vi "Main.vi"() -> ()   [LabVIEW 2017]
uses:
  <vilib>/Platform/TimedLoop/XDataNode/timing_clust.ctl
  <vilib>/Platform/TimedLoop/XDataNode/nitl_modes.ctl
  <vilib>/Platform/TimedLoop/XDataNode/wakeup.ctl
  <vilib>/Analysis/baseanly.llb/Mean (DBL).vi
  <vilib>/platform/TimedLoop/XDataNode/XDataNode.xnode
  <userlib>/dxl_x86_c/dxl_x86_c.lvlib
  <vilib>/Analysis/NI_AALBase.lvlib
  <vilib>/Platform/TimedLoop/XDataNode/XDNodeRunTimeDep.lvlib
panel:
  out "ADDR_MX_\nGOAL_POSITION":u16=30
  out "ADDR_MX_D":u16=26
  out "ADDR_MX_I":u16=27
  out "ADDR_MX_P":u16=28
  in  "PID gains":cluster{"Kp":dbl, "Ki":dbl, "Kd":dbl}={"Kp"=0.5, "Ki"=0.1, "Kd"=0.01} {"Kd" format="%.3f"; "Ki" format="%.3f"; "Kp" format="%.3f"}
  out "XY Graph":cluster{dbl[], dbl[]}(graph)={[0.0, 0.0, 21.21667205549289, 40.84932767864532, 14.13895464430464, 0.0], [0.0, 4.5, -15.269998150977838, -36.613822390853436, -25.31975437413041, 0.0]}
  in  "w":dbl=4.5
  in  "b 1":dbl=29.0
  in  "a 1":dbl=29.0
  out "theta 2":dbl=132.978515625
  out "theta 1":dbl=150.8203125
  out "delta load 2":dbl=0.09090909090908994
  out "value : MX\npresent speed 2":u16
  out "value : MX\npresent position 2":u16=2537
  out "value : MX\ngoal torque 2":u16
  out "value: MX\npresent load 2":u16=20
  in  "dynamixel_id 2":u8=11
  in  "locking ticks":i32=5
  in  "load trigger":dbl=40.0
  out "delta load 1":dbl=-2.8090909090909086
  out "value : MX\npresent speed 1":u16
  in  "torque 1 + torque 2":dbl=120.0
  out "CONTROL MODE":string="POSITION LOCK"
  out "value: MX\npresent load 1":u16=28
  out "ADDR_MX_\nPRESENT_LOAD":u16=40
  out "ADDR_MX_\nPRESENT_SPEED":u16=38
  out "ADDR_MX_\nTORQUE_CONTROL_MODE_ENABLE":u16=70
  out "value : MX\ngoal torque 1":u16
  in  "terminate":bool
  out "value : MX\npresent position 1":u16=2740
  out "baud_rate":i32=57600
  in  "dynamixel_id 1":u8=12
  out "protocol_version":dbl=1.0
  out "port_num":i32
  out "ADDR_MX_\nTORQUE_ENABLE":u16=24
  out "ADDR_MX_\nGOAL_TORQUE":u16=71
  out "ADDR_MX_\nPRESENT_POSITION":u16=36
  out "device_name":string="COM3"
  out "dynamixel_comm_result":string="[TxRxResult] Communication success."
  out "dynamixel_error":string
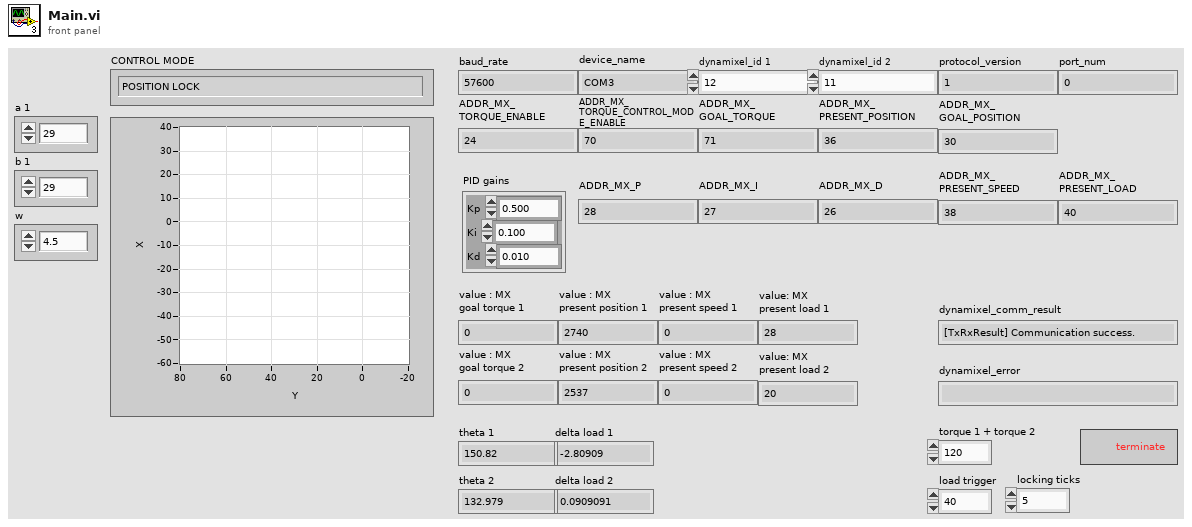
[diagram p1: front panel]
types:
  T1 = typedef "XDNodeRunTimeDep.lvlib/timing_clust.ctl" = cluster{"Expected End [f-1]":u64, "Actual End [f-1]":u64, "Finished Late? [f-1]":bool, "Expected End [i-1]":u64, "Actual End [i-1]":u64, "Finished Late? [i-1]":bool, "Expected Start [i]":u64, "Actual Start [i]":u64, "Expected Start [f]":u64, "Actual Start [f]":u64, "Source Name":string, "Structure Name":string, "Period":i64, "Deadline":i64, "Offset":i64, "Start":i64, "Priority":i32, "Timeout":i32, "Mode":T2, "Wakeup Reason":T3, "Error":errorcluster, "Source Type":string, "Secondary Source Type":string, "Global End Time":u64, "Global Start Time":u64, "Frame Duration":u64, "Iteration Duration":u64, "Assigned CPU":i32, "I/O Scan Engine Mode":u32}
  T2 = typedef "XDNodeRunTimeDep.lvlib/nitl_modes.ctl" = enum32{"No Change", "Process missed periods, maintain original phase", "Discard missed periods, maintain original phase", "Process missed periods, ignore original phase", "Discard missed periods, ignore original phase"}
  T3 = typedef "XDNodeRunTimeDep.lvlib/wakeup.ctl" = enum32{"Normal", "Aborted", "Asynchronous wakeup", "Timing source error", "Timed loop error", "Timeout"}
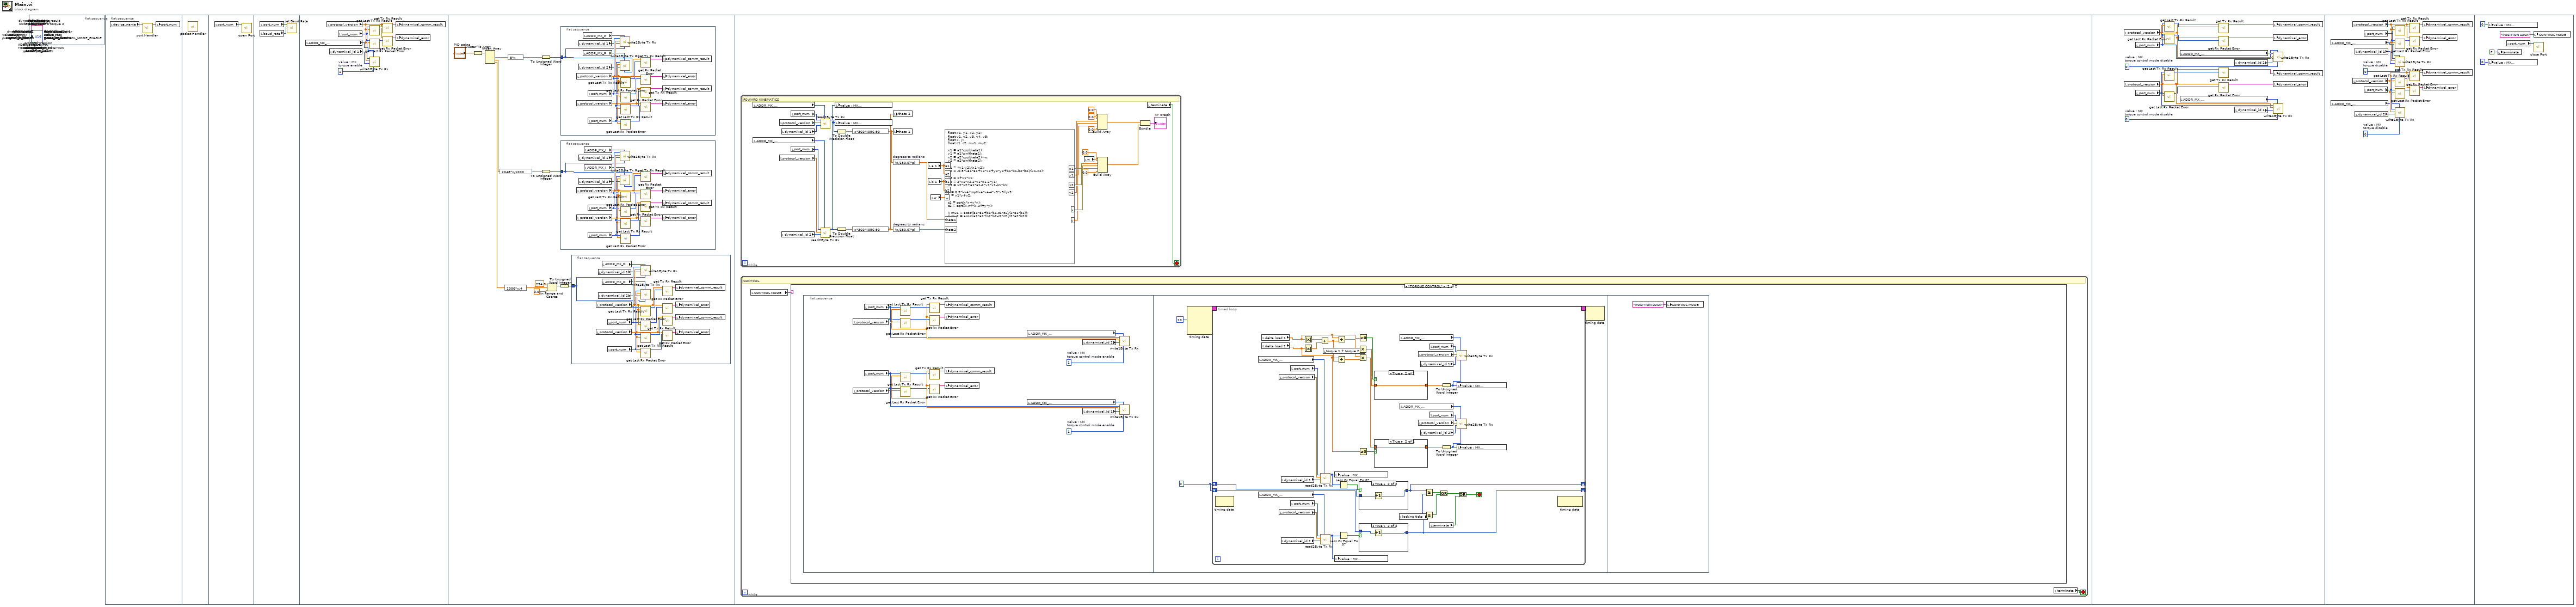
[diagram p0: block diagram]
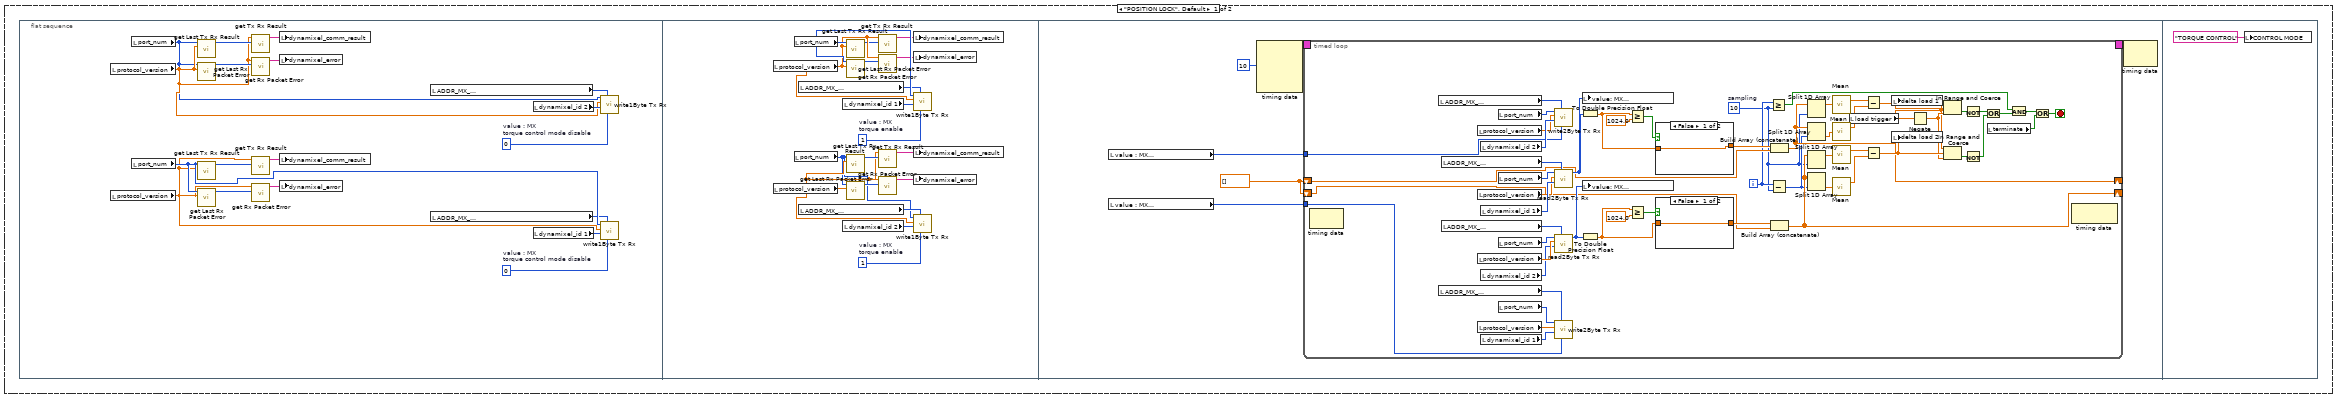
[diagram p2: hidden frame]
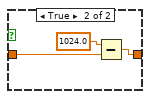
[diagram p3: hidden frame]
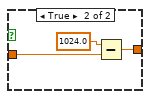
[diagram p4: hidden frame]
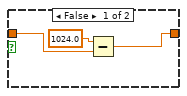
[diagram p5: hidden frame]
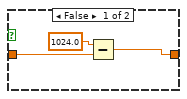
[diagram p6: hidden frame]
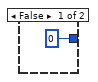
[diagram p7: hidden frame]
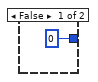
[diagram p8: hidden frame]
diagram:
  n1 = flat-sequence {
    frame #0 {
    }
  }
  n2 = flat-sequence {
    frame #0 {
      n3 = local read "device_name"() -> (w2:string)
      n4 = call <userlib>:"port Handler.vi"("port_name"=w2) -> ("function return"=w1:i32)  [unwired: 10 in]
      n5 = local write "port_num"(w1) -> ()
    }
    frame #1 {
      n6 = call <userlib>:"packet Handler.vi"() -> ()  [unwired: 12 in]
    }
    frame #2 {
      n7 = local read "port_num"() -> (w3:i32)
      n8 = call <userlib>:"open Port.vi"("port_num"=w3) -> ()  [unwired: 10 in, 1 out]
    }
    frame #3 {
      n9 = local read "port_num"() -> (w4:i32)
      n10 = local read "baud_rate"() -> (w5:i32)
      n11 = call <userlib>:"set Baud Rate.vi"("baudrate"=w5, "port_num"=w4) -> ()  [unwired: 9 in, 1 out]
    }
    frame #4 {
      w7 = 1  # value : MX torque enable
      n12 = local read "ADDR_MX_\nTORQUE_ENABLE"() -> (w14:u16)
      n13 = local read "protocol_version"() -> (w6:dbl)
      n14 = local read "dynamixel_id 1"() -> (w13:u8)
      n15 = local read "port_num"() -> (w8:i32)
      n16 = call <userlib>:"get Last Tx Rx Result.vi"("protocol_version"=w6, "port_num"=w8) -> ("function return"=w9:i32)  [unwired: 9 in]
      n17 = call <userlib>:"get Last Rx Packet Error.vi"("protocol_version"=w6, "port_num"=w8) -> ("function return"=w10:u8)  [unwired: 9 in]
      n18 = call <userlib>:"write1Byte Tx Rx.vi"("data"=w7, "address"=w14, "id"=w13, "protocol_version"=w6, "port_num"=w8) -> ()  [unwired: 7 in]
      n19 = call <userlib>:"get Tx Rx Result.vi"("result"=w9, "protocol_version"=w6) -> ("function return"=w11:string)  [unwired: 9 in]
      n20 = call <userlib>:"get Rx Packet Error.vi"("error"=w10, "protocol_version"=w6) -> ("function return"=w12:string)  [unwired: 9 in]
      n21 = local write "dynamixel_comm_result"(w11) -> ()
      n22 = local write "dynamixel_error"(w12) -> ()
    }
    frame #5 {
      n23 = Cluster To Array(cluster="PID gains") -> (array=w27:dbl[])
      n24 = Index Array(array=w27) -> (element #1=w26:dbl, element #2=w25:dbl, element #3=w24:dbl)  [unwired: 3 in]
      n25 = expression code="2048*x/1000"(w25) -> (w22:dbl)
      n26 = expression code="1000*x/4"(w24) -> (w19:dbl)
      n27 = expression code="8*x"(w26) -> (w23:dbl)
      n28 = To Unsigned Word Integer(number=w23) -> (unsigned 16bit integer=w17:u16)
      n29 = To Unsigned Word Integer(number=w22) -> (unsigned 16bit integer=w16:u16)
      n30 = In Range and Coerce(upper limit=254.0, x=w19, lower limit=0.0) -> (coerced(x)=w18:dbl)  [unwired: 1 out]
      n31 = To Unsigned Word Integer(number=w18) -> (unsigned 16bit integer=w15:u16)
      n32 = flat-sequence {
        tunnel: w17 -> [w63]
        frame #0 {
          n33 = local read "protocol_version"() -> (w79:dbl)
          n34 = local read "protocol_version"() -> (w64:dbl)
          n35 = local read "dynamixel_id 1"() -> (w73:u8)
          n36 = local read "dynamixel_id 2"() -> (w70:u8)
          n37 = local read "ADDR_MX_P"() -> (w72:u16)
          n38 = local read "ADDR_MX_P"() -> (w71:u16)
          n39 = local read "port_num"() -> (w78:i32)
          n40 = local read "port_num"() -> (w65:i32)
          n41 = call <userlib>:"write1Byte Tx Rx.vi"("data"=w63, "address"=w72, "id"=w73, "protocol_version"=w79, "port_num"=w78) -> ()  [unwired: 7 in]
          n42 = call <userlib>:"write1Byte Tx Rx.vi"("data"=w63, "address"=w71, "id"=w70, "protocol_version"=w64, "port_num"=w65) -> ()  [unwired: 7 in]
          n43 = call <userlib>:"get Last Tx Rx Result.vi"("protocol_version"=w79, "port_num"=w78) -> ("function return"=w77:i32)  [unwired: 9 in]
          n44 = call <userlib>:"get Last Rx Packet Error.vi"("protocol_version"=w79, "port_num"=w78) -> ("function return"=w76:u8)  [unwired: 9 in]
          n45 = call <userlib>:"get Last Tx Rx Result.vi"("protocol_version"=w64, "port_num"=w65) -> ("function return"=w66:i32)  [unwired: 9 in]
          n46 = call <userlib>:"get Last Rx Packet Error.vi"("protocol_version"=w64, "port_num"=w65) -> ("function return"=w67:u8)  [unwired: 9 in]
          n47 = call <userlib>:"get Tx Rx Result.vi"("result"=w77, "protocol_version"=w79) -> ("function return"=w75:string)  [unwired: 9 in]
          n48 = call <userlib>:"get Rx Packet Error.vi"("error"=w76, "protocol_version"=w79) -> ("function return"=w74:string)  [unwired: 9 in]
          n49 = call <userlib>:"get Tx Rx Result.vi"("result"=w66, "protocol_version"=w64) -> ("function return"=w68:string)  [unwired: 9 in]
          n50 = call <userlib>:"get Rx Packet Error.vi"("error"=w67, "protocol_version"=w64) -> ("function return"=w69:string)  [unwired: 9 in]
          n51 = local write "dynamixel_comm_result"(w75) -> ()
          n52 = local write "dynamixel_error"(w74) -> ()
          n53 = local write "dynamixel_comm_result"(w68) -> ()
          n54 = local write "dynamixel_error"(w69) -> ()
        }
      }
      n55 = flat-sequence {
        tunnel: w16 -> [w46]
        frame #0 {
          n56 = local read "protocol_version"() -> (w62:dbl)
          n57 = local read "protocol_version"() -> (w47:dbl)
          n58 = local read "dynamixel_id 1"() -> (w56:u8)
          n59 = local read "dynamixel_id 2"() -> (w53:u8)
          n60 = local read "ADDR_MX_I"() -> (w55:u16)
          n61 = local read "ADDR_MX_I"() -> (w54:u16)
          n62 = local read "port_num"() -> (w61:i32)
          n63 = local read "port_num"() -> (w48:i32)
          n64 = call <userlib>:"write1Byte Tx Rx.vi"("data"=w46, "address"=w55, "id"=w56, "protocol_version"=w62, "port_num"=w61) -> ()  [unwired: 7 in]
          n65 = call <userlib>:"write1Byte Tx Rx.vi"("data"=w46, "address"=w54, "id"=w53, "protocol_version"=w47, "port_num"=w48) -> ()  [unwired: 7 in]
          n66 = call <userlib>:"get Last Tx Rx Result.vi"("protocol_version"=w62, "port_num"=w61) -> ("function return"=w60:i32)  [unwired: 9 in]
          n67 = call <userlib>:"get Last Rx Packet Error.vi"("protocol_version"=w62, "port_num"=w61) -> ("function return"=w59:u8)  [unwired: 9 in]
          n68 = call <userlib>:"get Last Tx Rx Result.vi"("protocol_version"=w47, "port_num"=w48) -> ("function return"=w49:i32)  [unwired: 9 in]
          n69 = call <userlib>:"get Last Rx Packet Error.vi"("protocol_version"=w47, "port_num"=w48) -> ("function return"=w50:u8)  [unwired: 9 in]
          n70 = call <userlib>:"get Tx Rx Result.vi"("result"=w60, "protocol_version"=w62) -> ("function return"=w58:string)  [unwired: 9 in]
          n71 = call <userlib>:"get Rx Packet Error.vi"("error"=w59, "protocol_version"=w62) -> ("function return"=w57:string)  [unwired: 9 in]
          n72 = call <userlib>:"get Tx Rx Result.vi"("result"=w49, "protocol_version"=w47) -> ("function return"=w51:string)  [unwired: 9 in]
          n73 = call <userlib>:"get Rx Packet Error.vi"("error"=w50, "protocol_version"=w47) -> ("function return"=w52:string)  [unwired: 9 in]
          n74 = local write "dynamixel_comm_result"(w58) -> ()
          n75 = local write "dynamixel_error"(w57) -> ()
          n76 = local write "dynamixel_comm_result"(w51) -> ()
          n77 = local write "dynamixel_error"(w52) -> ()
        }
      }
      n78 = flat-sequence {
        tunnel: w15 -> [w29]
        frame #0 {
          n79 = local read "protocol_version"() -> (w45:dbl)
          n80 = local read "protocol_version"() -> (w30:dbl)
          n81 = local read "dynamixel_id 1"() -> (w39:u8)
          n82 = local read "dynamixel_id 2"() -> (w36:u8)
          n83 = local read "ADDR_MX_D"() -> (w38:u16)
          n84 = local read "ADDR_MX_D"() -> (w37:u16)
          n85 = local read "port_num"() -> (w44:i32)
          n86 = local read "port_num"() -> (w31:i32)
          n87 = call <userlib>:"write1Byte Tx Rx.vi"("data"=w29, "address"=w38, "id"=w39, "protocol_version"=w45, "port_num"=w44) -> ()  [unwired: 7 in]
          n88 = call <userlib>:"write1Byte Tx Rx.vi"("data"=w29, "address"=w37, "id"=w36, "protocol_version"=w30, "port_num"=w31) -> ()  [unwired: 7 in]
          n89 = call <userlib>:"get Last Tx Rx Result.vi"("protocol_version"=w45, "port_num"=w44) -> ("function return"=w43:i32)  [unwired: 9 in]
          n90 = call <userlib>:"get Last Rx Packet Error.vi"("protocol_version"=w45, "port_num"=w44) -> ("function return"=w42:u8)  [unwired: 9 in]
          n91 = call <userlib>:"get Last Tx Rx Result.vi"("protocol_version"=w30, "port_num"=w31) -> ("function return"=w32:i32)  [unwired: 9 in]
          n92 = call <userlib>:"get Last Rx Packet Error.vi"("protocol_version"=w30, "port_num"=w31) -> ("function return"=w33:u8)  [unwired: 9 in]
          n93 = call <userlib>:"get Tx Rx Result.vi"("result"=w43, "protocol_version"=w45) -> ("function return"=w41:string)  [unwired: 9 in]
          n94 = call <userlib>:"get Rx Packet Error.vi"("error"=w42, "protocol_version"=w45) -> ("function return"=w40:string)  [unwired: 9 in]
          n95 = call <userlib>:"get Tx Rx Result.vi"("result"=w32, "protocol_version"=w30) -> ("function return"=w34:string)  [unwired: 9 in]
          n96 = call <userlib>:"get Rx Packet Error.vi"("error"=w33, "protocol_version"=w30) -> ("function return"=w35:string)  [unwired: 9 in]
          n97 = local write "dynamixel_comm_result"(w41) -> ()
          n98 = local write "dynamixel_error"(w40) -> ()
          n99 = local write "dynamixel_comm_result"(w34) -> ()
          n100 = local write "dynamixel_error"(w35) -> ()
        }
      }
    }
    frame #6 {
      n101 = while {
        stop <- w81 stop-if-true
        # "FOWARD KINEMATICS"
        n102 = local read "ADDR_MX_\nPRESENT_POSITION"() -> (w114:u16)
        n103 = local read "ADDR_MX_\nPRESENT_POSITION"() -> (w107:u16)
        n104 = local read "protocol_version"() -> (w112:dbl)
        n105 = local read "protocol_version"() -> (w109:dbl)
        n106 = local read "dynamixel_id 1"() -> (w111:u8)
        n107 = local read "dynamixel_id 2"() -> (w110:u8)
        n108 = local read "port_num"() -> (w113:i32)
        n109 = local read "port_num"() -> (w108:i32)
        n110 = call <userlib>:"read2Byte Tx Rx.vi"("address"=w114, "id"=w111, "protocol_version"=w112, "port_num"=w113) -> ("function return"=w106:u16)  [unwired: 7 in]
        n111 = call <userlib>:"read2Byte Tx Rx.vi"("address"=w107, "id"=w110, "protocol_version"=w109, "port_num"=w108) -> ("function return"=w104:u16)  [unwired: 7 in]
        n112 = local write "value : MX\npresent position 2"(w104) -> ()
        n113 = local write "value : MX\npresent position 1"(w106) -> ()
        n114 = To Double Precision Float(number=w106) -> (double precision float=w105:dbl)
        n115 = To Double Precision Float(number=w104) -> (double precision float=w103:dbl)
        n116 = expression code="x*360/4096-90"(w105) -> (w88:dbl)
        n117 = expression code="x*360/4096-90"(w103) -> (w90:dbl)
        n118 = local write "theta 2"(w90) -> ()
        n119 = local write "theta 1"(w88) -> ()
        n120 = expression code="(x/180.0)*pi" "degrees to radians"(w88) -> (w87:dbl)
        n121 = expression code="(x/180.0)*pi" "degrees to radians"(w90) -> (w89:dbl)
        n122 = local read "a 1"() -> (w102:dbl)
        n123 = local read "b 1"() -> (w100:dbl)
        n124 = local read "w"() -> (w101:dbl)
        n125 = formula code="float x1, y1, x2, y2;\nfloat v1, v2, v3, v4, v5;\nfloat x, y;\nfloat c1, c2, mu1, mu2;\n\nx1 = a1*cos(theta1);\ny1 = a1*sin(theta1);\nx2 = a2*cos(theta2)+w;\ny2 = a2*sin(theta2);\n\nv1 = -(y1-y2)/(x1-x2);\nv2 = -0.5*(-a1*a1+x2*x2+y2*y2+b1*b1-b2*b2)/(x1-x2);\n\nv3 = 1+v1*v1;\nv4 = 2*v1*v2-2*v1*x1-2*y1;\nv5 = v2*v2+a1*a1-2*v2*x1-b1*b1;\n\ny = 0.5*(-v4+sqrt(v4*v4-4*v3*v5))/v3;\nx = v1*y+v2;\n\nc1 = sqrt(x*x+y*y);\nc2 = sqrt((x-w)*(x-w)+y*y);\n\n// mu1 = acos((a1*a1+b1*b1-c1*c1)/(2*a1*b1));\n// mu2 = acos((a2*a2+b2*b2-c2*c2)/(2*a2*b2));"("a1"=w102, "a2"=w102, "b1"=w100, "b2"=w100, "w"=w101, "theta1"=w87, "theta2"=w89) -> ("x1"=w96:dbl, "y1"=w93:dbl, "x2"=w98:dbl, "y2"=w95:dbl, "x"=w97:dbl, "y"=w94:dbl)
        n126 = local read "w"() -> (w99:dbl)
        n127 = Build Array(0.0 ("element"), 0.0 ("element"), w95, w94, w93, 0.0 ("element")) -> (w91:dbl[])
        n128 = Build Array(0.0 ("element"), w99, w98, w97, w96, 0.0 ("element")) -> (w92:dbl[])
        n129 = Bundle(w91, w92) -> (→"XY Graph":cluster{dbl[], dbl[]})  [unwired: 1 in]
        n130 = local read "terminate"() -> (w81:bool)
      }
      n131 = while {
        stop <- w116 stop-if-true
        # "CONTROL"
        n132 = local read "CONTROL MODE"() -> (w115:string)
        n133 = case shown="\"TORQUE CONTROL\"" w115 {
          frame "POSITION LOCK", Default {
            n134 = flat-sequence {
              frame #0 {
                w117 = 0  # value : MX torque control mode disable
                w134 = 0  # value : MX torque control mode disable
                n135 = local read "protocol_version"() -> (w119:dbl)
                n136 = local read "protocol_version"() -> (w132:dbl)
                n137 = local read "port_num"() -> (w118:i32)
                n138 = local read "port_num"() -> (w133:i32)
                n139 = call <userlib>:"get Last Tx Rx Result.vi"("protocol_version"=w119, "port_num"=w118) -> ("function return"=w120:i32)  [unwired: 9 in]
                n140 = call <userlib>:"get Last Rx Packet Error.vi"("protocol_version"=w119, "port_num"=w118) -> ("function return"=w121:u8)  [unwired: 9 in]
                n141 = call <userlib>:"get Last Tx Rx Result.vi"("protocol_version"=w132, "port_num"=w133) -> ("function return"=w131:i32)  [unwired: 9 in]
                n142 = call <userlib>:"get Last Rx Packet Error.vi"("protocol_version"=w132, "port_num"=w133) -> ("function return"=w130:u8)  [unwired: 9 in]
                n143 = call <userlib>:"get Tx Rx Result.vi"("result"=w120, "protocol_version"=w119) -> ("function return"=w122:string)  [unwired: 9 in]
                n144 = call <userlib>:"get Rx Packet Error.vi"("error"=w121, "protocol_version"=w119) -> ("function return"=w123:string)  [unwired: 9 in]
                n145 = call <userlib>:"get Tx Rx Result.vi"("result"=w131, "protocol_version"=w132) -> ("function return"=w129:string)  [unwired: 9 in]
                n146 = call <userlib>:"get Rx Packet Error.vi"("error"=w130, "protocol_version"=w132) -> ("function return"=w128:string)  [unwired: 9 in]
                n147 = local write "dynamixel_comm_result"(w122) -> ()
                n148 = local write "dynamixel_error"(w123) -> ()
                n149 = local write "dynamixel_comm_result"(w129) -> ()
                n150 = local write "dynamixel_error"(w128) -> ()
                n151 = local read "ADDR_MX_\nTORQUE_CONTROL_MODE_ENABLE"() -> (w125:u16)
                n152 = local read "ADDR_MX_\nTORQUE_CONTROL_MODE_ENABLE"() -> (w126:u16)
                n153 = local read "dynamixel_id 2"() -> (w124:u8)
                n154 = local read "dynamixel_id 1"() -> (w127:u8)
                n155 = call <userlib>:"write1Byte Tx Rx.vi"("data"=w117, "address"=w125, "id"=w124, "protocol_version"=w119, "port_num"=w118) -> ()  [unwired: 7 in]
                n156 = call <userlib>:"write1Byte Tx Rx.vi"("data"=w134, "address"=w126, "id"=w127, "protocol_version"=w132, "port_num"=w133) -> ()  [unwired: 7 in]
              }
              frame #1 {
                w135 = 1  # value : MX torque enable
                w152 = 1  # value : MX torque enable
                n157 = local read "protocol_version"() -> (w150:dbl)
                n158 = local read "protocol_version"() -> (w137:dbl)
                n159 = local read "port_num"() -> (w151:i32)
                n160 = local read "port_num"() -> (w136:i32)
                n161 = local read "ADDR_MX_\nTORQUE_ENABLE"() -> (w144:u16)
                n162 = local read "ADDR_MX_\nTORQUE_ENABLE"() -> (w143:u16)
                n163 = local read "dynamixel_id 1"() -> (w145:u8)
                n164 = local read "dynamixel_id 2"() -> (w142:u8)
                n165 = call <userlib>:"get Last Tx Rx Result.vi"("protocol_version"=w150, "port_num"=w151) -> ("function return"=w149:i32)  [unwired: 9 in]
                n166 = call <userlib>:"get Last Rx Packet Error.vi"("protocol_version"=w150, "port_num"=w151) -> ("function return"=w148:u8)  [unwired: 9 in]
                n167 = call <userlib>:"get Last Tx Rx Result.vi"("protocol_version"=w137, "port_num"=w136) -> ("function return"=w138:i32)  [unwired: 9 in]
                n168 = call <userlib>:"get Last Rx Packet Error.vi"("protocol_version"=w137, "port_num"=w136) -> ("function return"=w139:u8)  [unwired: 9 in]
                n169 = call <userlib>:"get Tx Rx Result.vi"("result"=w149, "protocol_version"=w150) -> ("function return"=w147:string)  [unwired: 9 in]
                n170 = call <userlib>:"get Rx Packet Error.vi"("error"=w148, "protocol_version"=w150) -> ("function return"=w146:string)  [unwired: 9 in]
                n171 = call <userlib>:"get Tx Rx Result.vi"("result"=w138, "protocol_version"=w137) -> ("function return"=w140:string)  [unwired: 9 in]
                n172 = call <userlib>:"get Rx Packet Error.vi"("error"=w139, "protocol_version"=w137) -> ("function return"=w141:string)  [unwired: 9 in]
                n173 = local write "dynamixel_comm_result"(w147) -> ()
                n174 = local write "dynamixel_error"(w146) -> ()
                n175 = call <userlib>:"write1Byte Tx Rx.vi"("data"=w152, "address"=w144, "id"=w145, "protocol_version"=w150, "port_num"=w151) -> ()  [unwired: 7 in]
                n176 = local write "dynamixel_comm_result"(w140) -> ()
                n177 = local write "dynamixel_error"(w141) -> ()
                n178 = call <userlib>:"write1Byte Tx Rx.vi"("data"=w135, "address"=w143, "id"=w142, "protocol_version"=w137, "port_num"=w136) -> ()  [unwired: 7 in]
              }
              frame #2 {
                w155 = dbl[] []
                n179 = local read "value : MX\npresent position 2"() -> (w154:u16)
                n180 = local read "value : MX\npresent position 1"() -> (w153:u16)
                n181 = node-c288(i64 10 ("Period")) -> (w158:T1)  [unwired: 3 in]
                n182 = timed-loop {
                  shift-right: [w180] -> _
                  shift-left: w155 -> [w206]
                  shift-right: [w185] -> _
                  shift-left: w155 -> [w191]
                  timing: w158 -> [_]
                  timing-out: [_] -> w157
                  tunnel: w154 -> [w160]
                  tunnel: w153 -> [w159]
                  i -> [w173]
                  stop <- w188 stop-if-true
                  w172 = 10  # sampling
                  n183 = node-c288() -> ()  [unwired: 1 in, 1 out]
                  n184 = local read "ADDR_MX_\nGOAL_POSITION"() -> (w164:u16)
                  n185 = local read "ADDR_MX_\nGOAL_POSITION"() -> (w165:u16)
                  n186 = local read "ADDR_MX_\nPRESENT_LOAD"() -> (w214:u16)
                  n187 = local read "ADDR_MX_\nPRESENT_LOAD"() -> (w192:u16)
                  n188 = local read "protocol_version"() -> (w162:dbl)
                  n189 = local read "protocol_version"() -> (w211:dbl)
                  n190 = local read "protocol_version"() -> (w195:dbl)
                  n191 = local read "protocol_version"() -> (w167:dbl)
                  n192 = local read "dynamixel_id 2"() -> (w163:u8)
                  n193 = local read "dynamixel_id 1"() -> (w212:u8)
                  n194 = local read "dynamixel_id 2"() -> (w194:u8)
                  n195 = local read "dynamixel_id 1"() -> (w166:u8)
                  n196 = local read "port_num"() -> (w161:i32)
                  n197 = local read "port_num"() -> (w213:i32)
                  n198 = local read "port_num"() -> (w193:i32)
                  n199 = local read "port_num"() -> (w168:i32)
                  n200 = call <userlib>:"write2Byte Tx Rx.vi"("data"=w160, "address"=w164, "id"=w163, "protocol_version"=w162, "port_num"=w161) -> ()  [unwired: 7 in]
                  n201 = call <userlib>:"read2Byte Tx Rx.vi"("address"=w214, "id"=w212, "protocol_version"=w211, "port_num"=w213) -> ("function return"=w207:u16)  [unwired: 7 in]
                  n202 = call <userlib>:"read2Byte Tx Rx.vi"("address"=w192, "id"=w194, "protocol_version"=w195, "port_num"=w193) -> ("function return"=w199:u16)  [unwired: 7 in]
                  n203 = call <userlib>:"write2Byte Tx Rx.vi"("data"=w159, "address"=w165, "id"=w166, "protocol_version"=w167, "port_num"=w168) -> ()  [unwired: 7 in]
                  n204 = To Double Precision Float(number=w207) -> (double precision float=w208:dbl)
                  n205 = To Double Precision Float(number=w199) -> (double precision float=w198:dbl)
                  n206 = local write "value: MX\npresent load 1"(w207) -> ()
                  n207 = local write "value: MX\npresent load 2"(w199) -> ()
                  n208 = Greater Or Equal?(x=w208, y=1024.0) -> (x >= y?=w209:bool)
                  n209 = Greater Or Equal?(x=w198, y=1024.0) -> (x >= y?=w197:bool)
                  n210 = case shown="False" w209 {
                    tunnel: w208 -> [w221 w223]
                    tunnel: [w221 w222] -> w204
                    frame False {
                    }
                    frame True {
                      n211 = Subtract(x=1024.0, y=w223) -> (x-y=w222:dbl)
                    }
                  }
                  n212 = case shown="False" w197 {
                    tunnel: w198 -> [w217 w219]
                    tunnel: [w217 w218] -> w201
                    frame False {
                    }
                    frame True {
                      n213 = Subtract(x=1024.0, y=w219) -> (x-y=w218:dbl)
                    }
                  }
                  n214 = Greater Or Equal?(x=w173, y=w172) -> (x >= y?=w174:bool)
                  n215 = Subtract(x=w173, y=w172) -> (x-y=w179:i32)
                  n216 = Build Array (concatenate)(w204, w206) -> (w180:dbl[])
                  n217 = Build Array (concatenate)(w201, w191) -> (w185:dbl[])
                  n218 = Split 1D Array(array=w180, index=w172) -> (first subarray=w205:dbl[])  [unwired: 1 out]
                  n219 = Split 1D Array(array=w180, index=w179) -> (second subarray=w181:dbl[])  [unwired: 1 out]
                  n220 = Split 1D Array(array=w185, index=w172) -> (first subarray=w200:dbl[])  [unwired: 1 out]
                  n221 = Split 1D Array(array=w185, index=w179) -> (second subarray=w186:dbl[])  [unwired: 1 out]
                  n222 = call-poly <vilib>:"Mean.vi"("X"=w205) -> ("mean"=w178:dbl)  [unwired: 1 out]
                  n223 = call-poly <vilib>:"Mean.vi"("X"=w181) -> ("mean"=w177:dbl)  [unwired: 1 out]
                  n224 = call-poly <vilib>:"Mean.vi"("X"=w200) -> ("mean"=w184:dbl)  [unwired: 1 out]
                  n225 = call-poly <vilib>:"Mean.vi"("X"=w186) -> ("mean"=w183:dbl)  [unwired: 1 out]
                  n226 = local read "load trigger"() -> (w169:dbl)
                  n227 = Subtract(x=w178, y=w177) -> (x-y=w176:dbl)
                  n228 = Subtract(x=w184, y=w183) -> (x-y=w182:dbl)
                  n229 = local write "delta load 1"(w176) -> ()
                  n230 = local write "delta load 2"(w182) -> ()
                  n231 = Negate(x=w169) -> (-x=w170:dbl)
                  n232 = In Range and Coerce(upper limit=w169, x=w176, lower limit=w170) -> (In Range?=w203:bool)  [unwired: 1 out]
                  n233 = In Range and Coerce(upper limit=w169, x=w182, lower limit=w170) -> (In Range?=w202:bool)  [unwired: 1 out]
                  n234 = Not(x=w203) -> (.not. x?=w187:bool)
                  n235 = Not(x=w202) -> (.not. x?=w190:bool)
                  n236 = Or(x=w187, y=w190) -> (x .or. y?=w175:bool)
                  n237 = local read "terminate"() -> (w189:bool)
                  n238 = And(x=w174, y=w175) -> (x .and. y?=w171:bool)
                  n239 = Or(x=w171, y=w189) -> (x .or. y?=w188:bool)
                  n240 = node-c288() -> ()  [unwired: 1 in, 1 out]
                }
                n241 = node-c288(w157) -> ()  [unwired: 1 out]
              }
              frame #3 {
                n242 = local write "CONTROL MODE"("TORQUE CONTROL" ("mode")) -> ()
              }
            }
          }
          frame "TORQUE CONTROL" {
            n243 = flat-sequence {
              frame #0 {
                w238 = 1  # value : MX torque control mode enable
                w239 = 1  # value : MX torque control mode enable
                n244 = local read "protocol_version"() -> (w231:dbl)
                n245 = local read "protocol_version"() -> (w246:dbl)
                n246 = local read "port_num"() -> (w230:i32)
                n247 = local read "port_num"() -> (w247:i32)
                n248 = call <userlib>:"get Last Tx Rx Result.vi"("protocol_version"=w231, "port_num"=w230) -> ("function return"=w232:i32)  [unwired: 9 in]
                n249 = call <userlib>:"get Last Rx Packet Error.vi"("protocol_version"=w231, "port_num"=w230) -> ("function return"=w233:u8)  [unwired: 9 in]
                n250 = call <userlib>:"get Last Tx Rx Result.vi"("protocol_version"=w246, "port_num"=w247) -> ("function return"=w245:i32)  [unwired: 9 in]
                n251 = call <userlib>:"get Last Rx Packet Error.vi"("protocol_version"=w246, "port_num"=w247) -> ("function return"=w244:u8)  [unwired: 9 in]
                n252 = call <userlib>:"get Tx Rx Result.vi"("result"=w232, "protocol_version"=w231) -> ("function return"=w234:string)  [unwired: 9 in]
                n253 = call <userlib>:"get Rx Packet Error.vi"("error"=w233, "protocol_version"=w231) -> ("function return"=w235:string)  [unwired: 9 in]
                n254 = call <userlib>:"get Tx Rx Result.vi"("result"=w245, "protocol_version"=w246) -> ("function return"=w243:string)  [unwired: 9 in]
                n255 = call <userlib>:"get Rx Packet Error.vi"("error"=w244, "protocol_version"=w246) -> ("function return"=w242:string)  [unwired: 9 in]
                n256 = local write "dynamixel_comm_result"(w234) -> ()
                n257 = local write "dynamixel_error"(w235) -> ()
                n258 = local write "dynamixel_comm_result"(w243) -> ()
                n259 = local write "dynamixel_error"(w242) -> ()
                n260 = local read "ADDR_MX_\nTORQUE_CONTROL_MODE_ENABLE"() -> (w237:u16)
                n261 = local read "ADDR_MX_\nTORQUE_CONTROL_MODE_ENABLE"() -> (w240:u16)
                n262 = local read "dynamixel_id 2"() -> (w236:u8)
                n263 = local read "dynamixel_id 1"() -> (w241:u8)
                n264 = call <userlib>:"write1Byte Tx Rx.vi"("data"=w238, "address"=w237, "id"=w236, "protocol_version"=w231, "port_num"=w230) -> ()  [unwired: 7 in]
                n265 = call <userlib>:"write1Byte Tx Rx.vi"("data"=w239, "address"=w240, "id"=w241, "protocol_version"=w246, "port_num"=w247) -> ()  [unwired: 7 in]
              }
              frame #1 {
                w251 = 0
                n266 = node-c288(i64 10 ("Period")) -> (w250:T1)  [unwired: 3 in]
                n267 = timed-loop {
                  shift-right: [w288] -> _
                  shift-left: w251 -> [w289]
                  shift-right: [w277] -> _
                  shift-left: w251 -> [w281]
                  timing: w250 -> [_]
                  timing-out: [_] -> w249
                  stop <- w291 stop-if-true
                  n268 = node-c288() -> ()  [unwired: 1 in, 1 out]
                  n269 = local read "ADDR_MX_\nPRESENT_SPEED"() -> (w297:u16)
                  n270 = local read "ADDR_MX_\nPRESENT_SPEED"() -> (w282:u16)
                  n271 = local read "delta load 1"() -> (w253:dbl)
                  n272 = local read "delta load 2"() -> (w252:dbl)
                  n273 = local read "protocol_version"() -> (w294:dbl)
                  n274 = local read "protocol_version"() -> (w285:dbl)
                  n275 = local read "dynamixel_id 1"() -> (w295:u8)
                  n276 = local read "dynamixel_id 2"() -> (w284:u8)
                  n277 = local read "port_num"() -> (w296:i32)
                  n278 = local read "port_num"() -> (w283:i32)
                  n279 = Absolute Value(x=w253) -> (abs(x)=w260:dbl)
                  n280 = Absolute Value(x=w252) -> (abs(x)=w261:dbl)
                  n281 = Add(x=w260, y=w261) -> (x+y=w259:dbl)
                  n282 = call <userlib>:"read2Byte Tx Rx.vi"("address"=w297, "id"=w295, "protocol_version"=w294, "port_num"=w296) -> ("function return"=w293:u16)  [unwired: 7 in]
                  n283 = call <userlib>:"read2Byte Tx Rx.vi"("address"=w282, "id"=w284, "protocol_version"=w285, "port_num"=w283) -> ("function return"=w286:u16)  [unwired: 7 in]
                  n284 = local read "torque 1 + torque 2"() -> (w256:dbl)
                  n285 = local write "value : MX\npresent speed 1"(w293) -> ()
                  n286 = local write "value : MX\npresent speed 2"(w286) -> ()
                  n287 = Divide(x=w253, y=w259) -> (x/y=w258:dbl)
                  n288 = Divide(x=w252, y=w259) -> (x/y=w257:dbl)
                  n289 = Less Or Equal To 0?(x=w293) -> (x <= 0?=w290:bool)
                  n290 = Less Or Equal To 0?(x=w286) -> (x <= 0?=w287:bool)
                  n291 = Multiply(x=w258, y=w256) -> (x*y=w254:dbl)
                  n292 = Multiply(x=w256, y=w257) -> (x*y=w255:dbl)
                  n293 = Greater Or Equal To 0?(x=w253) -> (x >= 0?=w275:bool)
                  n294 = Greater Or Equal To 0?(x=w252) -> (x >= 0?=w262:bool)
                  n295 = case shown="True" w290 {
                    tunnel: w289 -> [_ w313]
                    tunnel: [0 w312] -> w288
                    frame False {
                    }
                    frame True {
                      n296 = Increment(x=w313) -> (x+1=w312:i32)
                    }
                  }
                  n297 = case shown="True" w287 {
                    tunnel: w281 -> [_ w310]
                    tunnel: [0 w309] -> w277
                    frame False {
                    }
                    frame True {
                      n298 = Increment(x=w310) -> (x+1=w309:i32)
                    }
                  }
                  n299 = case shown="True" w275 {
                    tunnel: [w302 w305] -> w270
                    tunnel: w254 -> [w304 w305]
                    frame False {
                      n300 = Subtract(x=1024.0, y=w304) -> (x-y=w302:dbl)
                    }
                    frame True {
                    }
                  }
                  n301 = case shown="True" w262 {
                    tunnel: [w298 w301] -> w267
                    tunnel: w255 -> [w300 w301]
                    frame False {
                      n302 = Subtract(x=1024.0, y=w300) -> (x-y=w298:dbl)
                    }
                    frame True {
                    }
                  }
                  n303 = local read "locking ticks"() -> (w280:i32)
                  n304 = local read "ADDR_MX_\nGOAL_TORQUE"() -> (w271:u16)
                  n305 = local read "ADDR_MX_\nGOAL_TORQUE"() -> (w266:u16)
                  n306 = local read "protocol_version"() -> (w273:dbl)
                  n307 = local read "protocol_version"() -> (w264:dbl)
                  n308 = local read "dynamixel_id 1"() -> (w272:u8)
                  n309 = local read "dynamixel_id 2"() -> (w265:u8)
                  n310 = Greater Or Equal?(x=w288, y=w280) -> (x >= y?=w279:bool)
                  n311 = Greater Or Equal?(x=w277, y=w280) -> (x >= y?=w278:bool)
                  n312 = local read "port_num"() -> (w274:i32)
                  n313 = local read "port_num"() -> (w263:i32)
                  n314 = local read "terminate"() -> (w292:bool)
                  n315 = Or(x=w279, y=w278) -> (x .or. y?=w276:bool)
                  n316 = To Unsigned Word Integer(number=w270) -> (unsigned 16bit integer=w269:u16)
                  n317 = To Unsigned Word Integer(number=w267) -> (unsigned 16bit integer=w268:u16)
                  n318 = call <userlib>:"write2Byte Tx Rx.vi"("data"=w269, "address"=w271, "id"=w272, "protocol_version"=w273, "port_num"=w274) -> ()  [unwired: 7 in]
                  n319 = local write "value : MX\ngoal torque 1"(w269) -> ()
                  n320 = call <userlib>:"write2Byte Tx Rx.vi"("data"=w268, "address"=w266, "id"=w265, "protocol_version"=w264, "port_num"=w263) -> ()  [unwired: 7 in]
                  n321 = local write "value : MX\ngoal torque 2"(w268) -> ()
                  n322 = Or(x=w276, y=w292) -> (x .or. y?=w291:bool)
                  n323 = node-c288() -> ()  [unwired: 1 in, 1 out]
                }
                n324 = node-c288(w249) -> ()  [unwired: 1 out]
              }
              frame #2 {
                n325 = local write "CONTROL MODE"("POSITION LOCK" ("mode")) -> ()
              }
            }
          }
        }
        n326 = local read "terminate"() -> (w116:bool)
      }
    }
    frame #7 {
      w335 = 0  # value : MX torque control mode disable
      w320 = 0  # value : MX torque control mode disable
      n327 = local read "protocol_version"() -> (w329:dbl)
      n328 = local read "protocol_version"() -> (w326:dbl)
      n329 = local read "port_num"() -> (w328:i32)
      n330 = local read "port_num"() -> (w327:i32)
      n331 = call <userlib>:"get Last Tx Rx Result.vi"("protocol_version"=w329, "port_num"=w328) -> ("function return"=w330:i32)  [unwired: 9 in]
      n332 = call <userlib>:"get Last Rx Packet Error.vi"("protocol_version"=w329, "port_num"=w328) -> ("function return"=w331:u8)  [unwired: 9 in]
      n333 = call <userlib>:"get Last Tx Rx Result.vi"("protocol_version"=w326, "port_num"=w327) -> ("function return"=w325:i32)  [unwired: 9 in]
      n334 = call <userlib>:"get Last Rx Packet Error.vi"("protocol_version"=w326, "port_num"=w327) -> ("function return"=w324:u8)  [unwired: 9 in]
      n335 = local read "ADDR_MX_\nTORQUE_CONTROL_MODE_ENABLE"() -> (w336:u16)
      n336 = local read "ADDR_MX_\nTORQUE_CONTROL_MODE_ENABLE"() -> (w319:u16)
      n337 = call <userlib>:"get Tx Rx Result.vi"("result"=w330, "protocol_version"=w329) -> ("function return"=w332:string)  [unwired: 9 in]
      n338 = call <userlib>:"get Rx Packet Error.vi"("error"=w331, "protocol_version"=w329) -> ("function return"=w333:string)  [unwired: 9 in]
      n339 = call <userlib>:"get Tx Rx Result.vi"("result"=w325, "protocol_version"=w326) -> ("function return"=w323:string)  [unwired: 9 in]
      n340 = call <userlib>:"get Rx Packet Error.vi"("error"=w324, "protocol_version"=w326) -> ("function return"=w322:string)  [unwired: 9 in]
      n341 = local read "dynamixel_id 2"() -> (w334:u8)
      n342 = local read "dynamixel_id 1"() -> (w321:u8)
      n343 = local write "dynamixel_comm_result"(w332) -> ()
      n344 = local write "dynamixel_error"(w333) -> ()
      n345 = call <userlib>:"write1Byte Tx Rx.vi"("data"=w335, "address"=w336, "id"=w334, "protocol_version"=w329, "port_num"=w328) -> ()  [unwired: 7 in]
      n346 = local write "dynamixel_comm_result"(w323) -> ()
      n347 = local write "dynamixel_error"(w322) -> ()
      n348 = call <userlib>:"write1Byte Tx Rx.vi"("data"=w320, "address"=w319, "id"=w321, "protocol_version"=w326, "port_num"=w327) -> ()  [unwired: 7 in]
    }
    frame #8 {
      w338 = 0  # value : MX torque disable
      w353 = 0  # value : MX torque disable
      n349 = local read "ADDR_MX_\nTORQUE_ENABLE"() -> (w354:u16)
      n350 = local read "ADDR_MX_\nTORQUE_ENABLE"() -> (w337:u16)
      n351 = local read "protocol_version"() -> (w347:dbl)
      n352 = local read "protocol_version"() -> (w344:dbl)
      n353 = local read "dynamixel_id 1"() -> (w352:u8)
      n354 = local read "dynamixel_id 2"() -> (w339:u8)
      n355 = local read "port_num"() -> (w346:i32)
      n356 = local read "port_num"() -> (w345:i32)
      n357 = call <userlib>:"get Last Tx Rx Result.vi"("protocol_version"=w347, "port_num"=w346) -> ("function return"=w348:i32)  [unwired: 9 in]
      n358 = call <userlib>:"get Last Rx Packet Error.vi"("protocol_version"=w347, "port_num"=w346) -> ("function return"=w349:u8)  [unwired: 9 in]
      n359 = call <userlib>:"write1Byte Tx Rx.vi"("data"=w353, "address"=w354, "id"=w352, "protocol_version"=w347, "port_num"=w346) -> ()  [unwired: 7 in]
      n360 = call <userlib>:"get Last Tx Rx Result.vi"("protocol_version"=w344, "port_num"=w345) -> ("function return"=w343:i32)  [unwired: 9 in]
      n361 = call <userlib>:"get Last Rx Packet Error.vi"("protocol_version"=w344, "port_num"=w345) -> ("function return"=w342:u8)  [unwired: 9 in]
      n362 = call <userlib>:"write1Byte Tx Rx.vi"("data"=w338, "address"=w337, "id"=w339, "protocol_version"=w344, "port_num"=w345) -> ()  [unwired: 7 in]
      n363 = call <userlib>:"get Tx Rx Result.vi"("result"=w348, "protocol_version"=w347) -> ("function return"=w350:string)  [unwired: 9 in]
      n364 = call <userlib>:"get Rx Packet Error.vi"("error"=w349, "protocol_version"=w347) -> ("function return"=w351:string)  [unwired: 9 in]
      n365 = call <userlib>:"get Tx Rx Result.vi"("result"=w343, "protocol_version"=w344) -> ("function return"=w341:string)  [unwired: 9 in]
      n366 = call <userlib>:"get Rx Packet Error.vi"("error"=w342, "protocol_version"=w344) -> ("function return"=w340:string)  [unwired: 9 in]
      n367 = local write "dynamixel_comm_result"(w350) -> ()
      n368 = local write "dynamixel_error"(w351) -> ()
      n369 = local write "dynamixel_comm_result"(w341) -> ()
      n370 = local write "dynamixel_error"(w340) -> ()
    }
    frame #9 {
      n371 = local write "value : MX\ngoal torque 2"(u16 0 ("value : MX (dial)\ngoal torque")) -> ()
      n372 = local write "value : MX\ngoal torque 1"(u16 0 ("value : MX (dial)\ngoal torque")) -> ()
      n373 = local write "terminate"(FALSE ("terminate")) -> ()
      n374 = local read "port_num"() -> (w359:i32)
      n375 = local write "CONTROL MODE"("POSITION LOCK" ("mode")) -> ()
      n376 = call <userlib>:"close Port.vi"("port_num"=w359) -> ()  [unwired: 11 in]
    }
  }
